vi "Read Valid Messages.vi"(8 "error in (no error)":errorcluster, 11 "controller in":refnum<class "Generic Plugin.lvclass">) -> (0 "error out":errorcluster, 2 "Valid Messages":string[](array[string]), 3 "controller out":refnum<class "Generic Plugin.lvclass">)   [LabVIEW 2020, in "Generic Plugin.lvclass"]
uses:
  Generic Plugin.lvclass
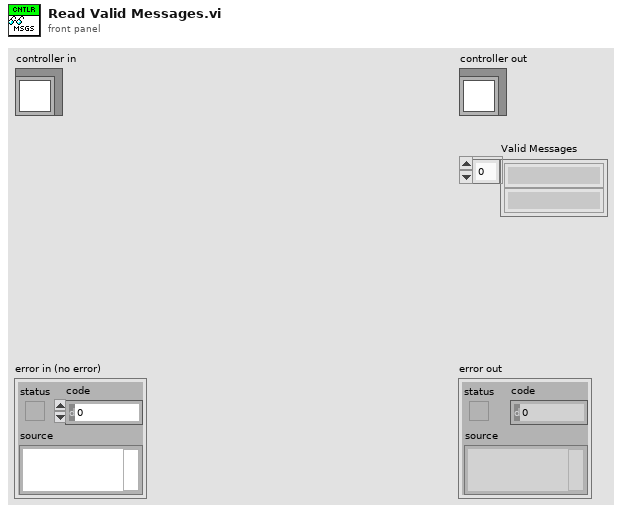
[diagram p1: front panel]
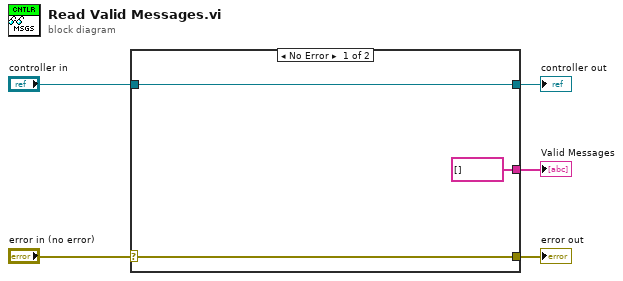
[diagram p0: block diagram]
diagram:
  n1 = case shown="No Error" "error in (no error)" {
    selector: "error in (no error)" -> [w8 w9]
    tunnel: [w8 w9] -> w4
    tunnel: [w7 w10] -> w2
    tunnel: "controller in" -> [w7 w10]
    tunnel: [string[] [] ("Valid Messages") _] -> w1
    frame No Error {
    }
    frame Error {
    }
  }
  "error out" <- w4
  "controller out" <- w2
  "Valid Messages" <- w1
